vi "command write-read placa.vi"(0 "Write Command":string, 2 "COM DATA":T1={"IP "="192.168.1.7", "Puerto:"=2101, "Time Out"=500}, 3 "bytes":u16) -> (5 "data out":string, 7 "error out":errorcluster)   [LabVIEW 2010]
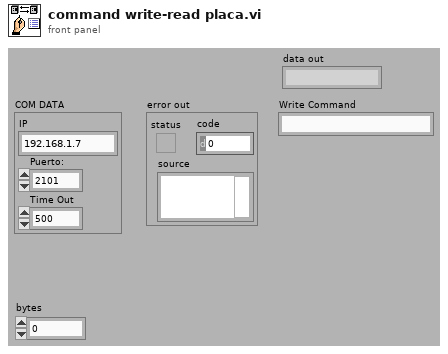
[diagram p1: front panel]
types:
  T1 = cluster{"IP ":string, "Puerto:":u16, "Time Out":u16}
  T2 = cluster{"connection ID":refnum<k5>, "Time Out":u16, "error out":errorcluster}
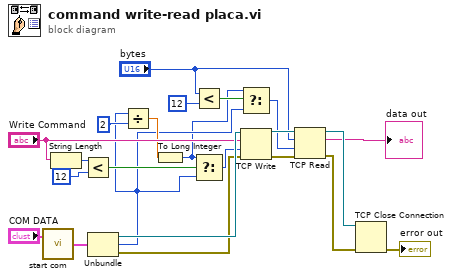
[diagram p0: block diagram]
diagram:
  n1 = call "start com.vi"("COM DATA"="COM DATA") -> ("ONLINE OUT"=w19:T2)  [unwired: 1 in]
  n2 = String Length(string="Write Command") -> (length=w13:i32)
  n3 = Less?(x=w13, y=12) -> (x < y?=w11:bool)
  n4 = Unbundle(w19) -> ("connection ID"=w17:refnum<k5>, "Time Out"=w4:u16, "error out"=w16:errorcluster)
  n5 = Divide(x=w4, y=u16 2) -> (x/y=w8:dbl)
  n6 = To Long Integer(number=w8) -> (32bit integer=w3:i32)
  n7 = Less?(x="bytes", y=12) -> (x < y?=w6:bool)
  n8 = Select(t=w3, s=w11, f=w4) -> (s? t:f=w10:i32)
  n9 = Select(t=w3, s=w6, f=w4) -> (s? t:f=w5:i32)
  n10 = TCP Write(connection ID=w17, data in="Write Command", error in (no error)=w16, 9:w10) -> (connection ID out=w23:refnum<k5>, error out=w22:errorcluster)  [unwired: 1 out]
  n11 = TCP Read(connection ID=w23, bytes to read="bytes", error in (no error)=w22, 9:w5) -> (connection ID out=w20:refnum<k5>, data out=→"data out":string, error out=w15:errorcluster)  [unwired: 1 in]
  n12 = TCP Close Connection(connection ID=w20, error in (no error)=w15) -> (error out=→"error out":errorcluster)  [unwired: 1 in, 1 out]
